vi "Write Number of Columns.vi"(5 "Number of Columns":u32, 9 "Array in":refnum<class "Array.lvclass">) -> (3 "Array out":refnum<class "Array.lvclass">)   [LabVIEW 2014, in "Array.lvclass"]
uses:
  Array.lvclass
  Array.lvclass/Array.ctl
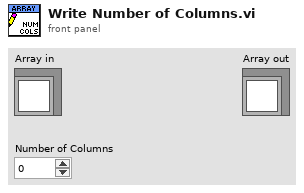
[diagram p1: front panel]
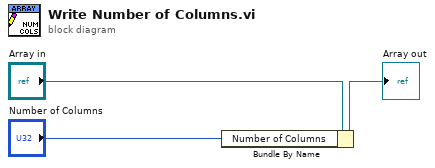
[diagram p0: block diagram]
diagram:
  n1 = Bundle By Name(cluster="Array in", "Number of Columns"="Number of Columns") -> (→"Array out":refnum<class "Array.lvclass">)
